vi "Inlet Convert Temp to Volt.vi"(7 "Inlet Temperature":dbl, 11 "Error In":errorcluster) -> (8 "Inlet Voltage":dbl, 15 "Error Out":errorcluster)   [LabVIEW 2016]
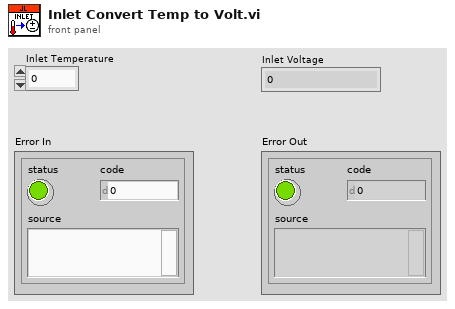
[diagram p1: front panel]
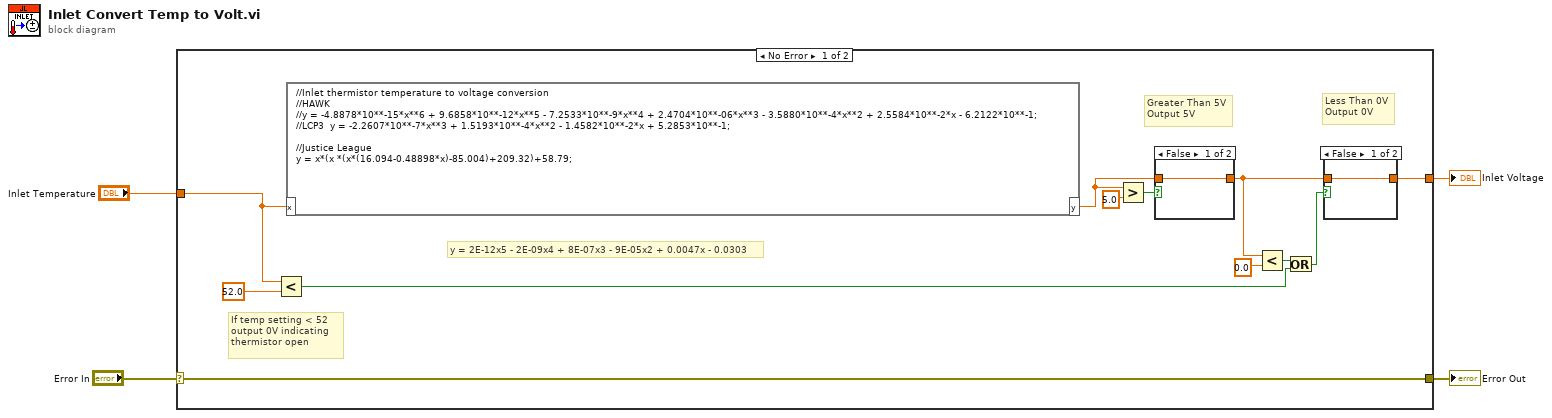
[diagram p0: block diagram]
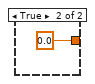
[diagram p2: hidden frame]
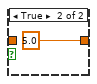
[diagram p3: hidden frame]
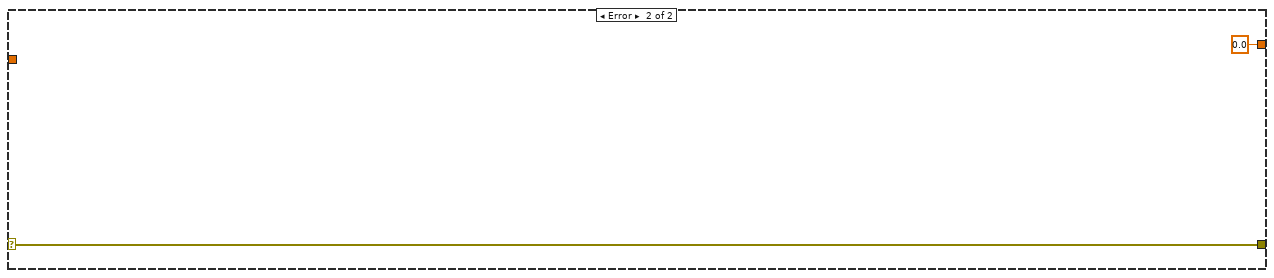
[diagram p4: hidden frame]
diagram:
  n1 = case shown="No Error" "Error In" {
    selector: "Error In" -> [w5 w21]
    tunnel: [w12 0.0 ("y")] -> w4
    tunnel: "Inlet Temperature" -> [w8 _]
    tunnel: [w5 w21] -> w1
    frame No Error {
      # "y = 2E-12x5 - 2E-09x4 + 8E-07x3 - 9E-05x2 + 0.0047x - 0.0303"
      # "Greater Than 5V\nOutput 5V"
      # "Less Than 0V\nOutput 0V"
      # "If temp setting < 52 \noutput 0V indicating \nthermistor open"
      n2 = Less?(x=w8, y=52.0) -> (x < y?=w6:bool)
      n3 = formula code="//Inlet thermistor temperature to voltage conversion\n//HAWK\n//y = -4.8878*10**-15*x**6 + 9.6858*10**-12*x**5 - 7.2533*10**-9*x**4 + 2.4704*10**-06*x**3 - 3.5880*10**-4*x**2 + 2.5584*10**-2*x - 6.2122*10**-1;\n//LCP3  y = -2.2607*10**-7*x**3 + 1.5193*10**-4*x**2 - 1.4582*10**-2*x + 5.2853*10**-1;\n\n//Justice League\ny = x*(x *(x*(16.094-0.48898*x)-85.004)+209.32)+58.79;"("x"=w8) -> ("y"=w15:dbl)
      n4 = Greater?(x=w15, y=5.0) -> (0:w13:bool)
      n5 = case shown="False" w13 {
        tunnel: [w19 5.0 ("y")] -> w11
        tunnel: w15 -> [w19 _]
        frame False {
        }
        frame True {
        }
      }
      n6 = Less?(x=w11, y=0.0) -> (x < y?=w10:bool)
      n7 = Or(x=w10, y=w6) -> (x .or. y?=w9:bool)
      n8 = case shown="False" w9 {
        tunnel: [w17 0.0 ("y")] -> w12
        tunnel: w11 -> [w17 _]
        frame False {
        }
        frame True {
        }
      }
    }
    frame Error {
    }
  }
  "Inlet Voltage" <- w4
  "Error Out" <- w1
